vi "RSZVB Select S-Parameters.vi"(6 "Out Port (1)":i32=1, 7 "In Port (1)":i32=1, 8 "error in (no error)":errorcluster {"code" format="%.0x"}, 9 "Trace Name (Trc1)":string="Trc1", 10 "Channel (1)":i32=1, 11 "VISA session":refnum<visa-resource-name>) -> (0 "error out":errorcluster {"code" format="%.0x"}, 3 "dup VISA session":refnum<visa-resource-name>)   [LabVIEW 2015]
doc: "This VI select one of the four elements of the standard 2-port scattering matrix (S-parameters) or select S-parameters for multiport measurements.\n\nAssigns a measurement parameter to an existing trace or creates a trace and assigns a channel number, a name and a measurement parameter to it. The trace is not displayed.\n\nThe S-parameters are the basic measured quantities of a network analyzer. They describe how the DUT modifies a signal that is transmitted or reflected in forward or reverse direction. S-parameters are expressed as S<out><in>, where <out> and <in> denote the output and input port numbers of the DUT.\n\nRemote-control command(s):\nCALCulate<Ch>:PARameter:SDEFine '<string>', 'S11' | 'S12' | 'S21' | 'S22' | ...\nCALCulate<Ch>:PARameter:MEASure '<string>', 'S11' | 'S12' | 'S21' | 'S22' | ..."
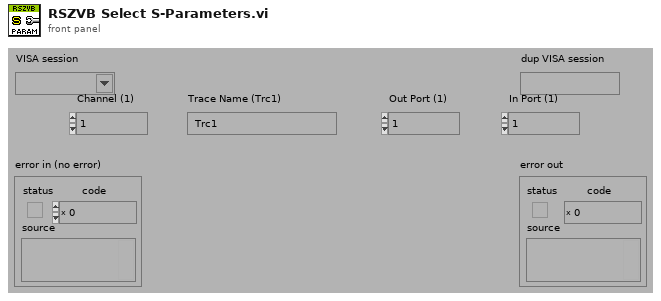
[diagram p1: front panel]
types:
  T1 = cluster{"Error Checking (T: On)":bool, "Installed Options":string[], "Data Valid?":bool, "Ports":i32, "Model":string[], "Option Checking (T: On)":bool}
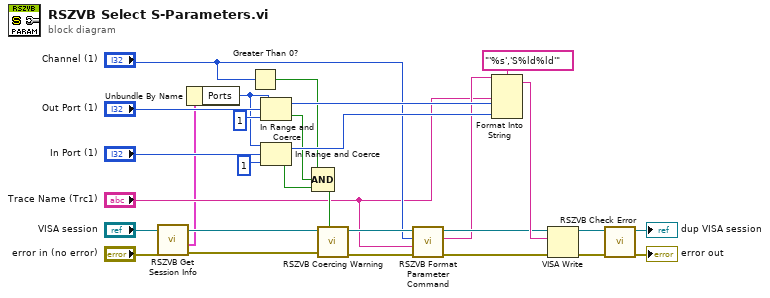
[diagram p0: block diagram]
diagram:
  n1 = call "RSZVB Get Session Info.vi"("error in (no error)"="error in (no error)", "VISA session"="VISA session") -> ("error out"=w3:errorcluster, "Session Info"=w2:T1, "dup VISA session"=w5:refnum<visa-resource-name>)  [unwired: 7 in]
  n2 = Unbundle By Name(w2) -> ("Ports"=w1:i32)
  n3 = Greater Than 0?(x="Channel (1)") -> (x > 0?=w23:bool)
  n4 = In Range and Coerce(upper limit=w1, x="Out Port (1)", lower limit=1) -> (coerced(x)=w24:i32, In Range?=w8:bool)
  n5 = In Range and Coerce(upper limit=w1, x="In Port (1)", lower limit=1) -> (coerced(x)=w28:i32, In Range?=w7:bool)
  n6 = Compound Arithmetic op=AND(w23, w8, w7) -> (w22:bool)
  n7 = call "RSZVB Coercing Warning.vi"("In Range?"=w22, "error in (no error)"=w3, "VISA session"=w5) -> ("error out"=w17:errorcluster, "dup VISA session"=w16:refnum<visa-resource-name>)  [unwired: 7 in]
  n8 = call "RSZVB Format Parameter Command.vi"("error in (no error)"=w17, "Trace Name (Trc1)"="Trace Name (Trc1)", "Channel (1)"="Channel (1)", "VISA session"=w16) -> ("error out"=w18:errorcluster, "Buffer"=w10:string, "dup VISA session"=w15:refnum<visa-resource-name>)  [unwired: 5 in]
  n9 = Format Into String(format string="'%s','S%ld%ld'", initial string=w10, "Trace Name (Trc1)", w24, w28) -> (resulting string=w21:string)  [unwired: 1 in, 1 out]
  n10 = VISA Write(VISA resource name=w15, write buffer=w21, error in (no error)=w18) -> (VISA resource name out=w25:refnum<visa-resource-name>, error out=w26:errorcluster)  [unwired: 1 out]
  n11 = call "RSZVB Check Error.vi"("error in (no error)"=w26, "VISA session"=w25) -> ("error out"=→"error out":errorcluster, "dup VISA session"=→"dup VISA session":refnum<visa-resource-name>)  [unwired: 8 in]
